vi "rsidr_core_global.vi"() -> ()   [LabVIEW 2020, in "Rohde&Schwarz RTx Oscilloscopes.lvlib"]
doc: "This Global variable contains driver's:\n- Attributes\n- Range Tables\n- Repeated Capabilities"
uses:
  Rohde&Schwarz RTx Oscilloscopes.lvlib
  type_Input_Format_Attribute.ctl
  type_Input_Format_RangeTable.ctl
  type_Input_Format_RepCap.ctl
  rsidr_core.lvlib
panel:
  in  "Repeated Capabilities":T1[](array[typedef])=[{"repCapName"="Channel", "indetifiers"=["CH0", "CH1", "CH2", "CH3", "CH4", "CHExt"], "cmdValues"=["", "1", "2", "3", "4", "5"]}, {"repCapName"="Measurement", "indetifiers"=["M1", "M2", "M3", "M4", "M5", "M6", "M7", "M8"], "cmdValues"=["1", "2", "3", "4", "5", "6", "7", "8"]}, {"repCapName"="Math", "indetifiers"=["MA1", "MA2", "MA3", "MA4", "MA5"], "cmdValues"=["1", "2", "3", "4", "5"]}, {"repCapName"="ReferenceWfm", "indetifiers"=["RW1", "RW2", "RW3", "RW4"], "cmdValues"=["1", "2", "3", "4"]}, {"repCapName"="SerialBus", "indetifiers"=["SB1", "SB2", "SB3", "SB4"], "cmdValues"=["1", "2", "3", "4"]}, {"repCapName"="Cursor", "indetifiers"=["Cur1", "Cur2", "Cur3"], "cmdValues"=["1", "2", "3"]}, {"repCapName"="ResultNumber", "indetifiers"=["Res1", "Res2", "Res3", "Res4", "Res5", "Res6", "Res7", "Res8", "Res9", "Res10", "Res11", "Res12", "Res13", "Res14", "Res15", "Res16", "Res17", "Res18", "Res19", "Res20", "Res21", "Res22", "Res23", "Res24", "Res25", "Res26", "Res27", "Res28", "Res29", "Res30", "Res31", "Res32", "Res33", "Res34", "Res35", "Res36", "Res37", "Res38", "Res39", "Res40"], "cmdValues"=["1", "2", "3", "4", "5", "6", "7", "8", "9", "10", "11", "12", "13", "14", "15", "16", "17", "18", "19", "20", "21", "22", "23", "24", "25", "26", "27", "28", "29", "30", "31", "32", "33", "34", "35", "36", "37", "38", "39", "40"]}, {"repCapName"="Gate", "indetifiers"=["Gate1", "Gate2", "Gate3"], "cmdValues"=["1", "2", "3"]}, {"repCapName"="OnOffResult", "indetifiers"=["OOR1", "OOR2", "OOR3"], "cmdValues"=["1", "2", "3"]}, {"repCapName"="SourceNumber", "indetifiers"=["S1", "S2", "S3", "S4"], "cmdValues"=["1", "2", "3", "4"]}, {"repCapName"="TDMChannel", "indetifiers"=["TDM0", "TDM1", "TDM2", "TDM3", "TDM4", "TDM5", "TDM6", "TDM7", "TDM8"], "cmdValues"=["", "1", "2", "3", "4", "5", "6", "7", "8"]}, {"repCapName"="Digital", "indetifiers"=["D0", "D1", "D2", "D3", "D4", "D5", "D6", "D7", "D8", "D9", "D10", "D11", "D12", "D13", "D14", "D15"], "cmdValues"=["0", "1", "2", "3", "4", "5", "6", "7", "8", "9", "10", "11", "12", "13", "14", "15"]}, {"repCapName"="DigitalVoltmeter", "indetifiers"=["DVM1", "DVM2", "DVM3", "DVM4"], "cmdValues"=["1", "2", "3", "4"]}, {"repCapName"="CursorLine", "indetifiers"=["CursorLine1", "CursorLine2"], "cmdValues"=["1", "2"]}, {"repCapName"="Logic", "indetifiers"=["Logic1", "Logic2"], "cmdValues"=["1", "2"]}, {"repCapName"="OutputPin", "indetifiers"=["P0", "P1", "P2", "P3"], "cmdValues"=["0", "1", "2", "3"]}, {"repCapName"="ProfilePoint", "indetifiers"=["Point1", "Point2", "Point3", "Point4", "Point5", "Point6", "Point7", "Point8", "Point9", "Point10", "Point11", "Point12", "Point13", "Point14", "Point15", "Point16"], "cmdValues"=["1", "2", "3", "4", "5", "6", "7", "8", "9", "10", "11", "12", "13", "14", "15", "16"]}, {"repCapName"="BodeMarker", "indetifiers"=["BodeMark1", "BodeMark2"], "cmdValues"=["1", "2"]}, {"repCapName"="ParallelLine", "indetifiers"=["Bit0", "Bit1", "Bit2", "Bit3", "Bit4", "Bit5", "Bit6", "Bit7", "Bit8", "Bit9", "Bit10", "Bit11", "Bit12", "Bit13", "Bit14", "Bit15"], "cmdValues"=["0", "1", "2", "3", "4", "5", "6", "7", "8", "9", "10", "11", "12", "13", "14", "15"]}]
  in  "Range Tables":T2[](array[typedef])=[{"Type"=0, "Name"="rsrtx_rngHorzScale", "Entries"=[{"Name"="", "Value 1"=1e-09, "Value 2"=50.0, "Command"=""}]}, {"Type"=0, "Name"="rsrtx_rngHorzAcquisitionTime", "Entries"=[{"Name"="", "Value 1"=2.5e-10, "Value 2"=500.0, "Command"=""}]}, {"Type"=0, "Name"="rsrtx_rngAcquisitionStartTime", "Entries"=[{"Name"="", "Value 1"=-500.0, "Value 2"=500.0, "Command"=""}]}, {"Type"=0, "Name"="rsrtx_rngHorzReference", "Entries"=[{"Name"="", "Value 1"=8.33, "Value 2"=91.67, "Command"=""}]}, {"Type"=2, "Name"="rsrtx_rngSampleMode", "Entries"=[{"Name"="Real Time", "Value 1"=0.0, "Value 2"=0.0, "Command"="RTIM"}, {"Name"="Equivalent Time", "Value 1"=1.0, "Value 2"=0.0, "Command"="ETIM"}]}, {"Type"=2, "Name"="rsrtx_rngWaveformArithmetics", "Entries"=[{"Name"="Off", "Value 1"=0.0, "Value 2"=0.0, "Command"="OFF"}, {"Name"="Envelope", "Value 1"=1.0, "Value 2"=0.0, "Command"="ENV"}, {"Name"="Average", "Value 1"=2.0, "Value 2"=0.0, "Command"="AVER"}, {"Name"="Smooth", "Value 1"=3.0, "Value 2"=0.0, "Command"="SMO"}, {"Name"="Filter", "Value 1"=4.0, "Value 2"=0.0, "Command"="FILT"}]}, {"Type"=2, "Name"="rsrtx_rngVerticalCoupling", "Entries"=[{"Name"="AC", "Value 1"=0.0, "Value 2"=0.0, "Command"="AC"}, {"Name"="DC 50 Ohm", "Value 1"=1.0, "Value 2"=0.0, "Command"="DC"}, {"Name"="DC 1 MOhm", "Value 1"=2.0, "Value 2"=0.0, "Command"="DCL"}, {"Name"="AC 1 MOhm", "Value 1"=3.0, "Value 2"=0.0, "Command"="ACL"}, {"Name"="Ground", "Value 1"=4.0, "Value 2"=0.0, "Command"="GND"}]}, {"Type"=2, "Name"="rsrtx_rngChannelBWLimit", "Entries"=[{"Name"="Full", "Value 1"=0.0, "Value 2"=0.0, "Command"="FULL"}, {"Name"="400 MHz", "Value 1"=1.0, "Value 2"=0.0, "Command"="B400"}, {"Name"="200 MHz", "Value 1"=2.0, "Value 2"=0.0, "Command"="B200"}, {"Name"="20 MHz", "Value 1"=3.0, "Value 2"=0.0, "Command"="B20"}]}, {"Type"=2, "Name"="rsrtx_rngTriggerSource", "Entries"=[{"Name"="Channel 1", "Value 1"=1.0, "Value 2"=0.0, "Command"="CH1"}, {"Name"="Channel 2", "Value 1"=2.0, "Value 2"=0.0, "Command"="CH2"}, {"Name"="Channel 3", "Value 1"=3.0, "Value 2"=0.0, "Command"="CH3"}, {"Name"="Channel 4", "Value 1"=4.0, "Value 2"=0.0, "Command"="CH4"}, {"Name"="External Trigger Input", "Value 1"=5.0, "Value 2"=0.0, "Command"="EXT"}, {"Name"="AC Line", "Value 1"=6.0, "Value 2"=0.0, "Command"="LINE"}, {"Name"="Serial Bus 1", "Value 1"=7.0, "Value 2"=0.0, "Command"="SBUS1"}, {"Name"="Serial Bus 2", "Value 1"=8.0, "Value 2"=0.0, "Command"="SBUS2"}, {"Name"="Serial Bus 3", "Value 1"=9.0, "Value 2"=0.0, "Command"="SBUS3"}, {"Name"="Serial Bus 4", "Value 1"=10.0, "Value 2"=0.0, "Command"="SBUS4"}, {"Name"="Digital 0", "Value 1"=11.0, "Value 2"=0.0, "Command"="D0"}, {"Name"="Digital 1", "Value 1"=12.0, "Value 2"=0.0, "Command"="D1"}, {"Name"="Digital 2", "Value 1"=13.0, "Value 2"=0.0, "Command"="D2"}, {"Name"="Digital 3", "Value 1"=14.0, "Value 2"=0.0, "Command"="D3"}, {"Name"="Digital 4", "Value 1"=15.0, "Value 2"=0.0, "Command"="D4"}, {"Name"="Digital 5", "Value 1"=16.0, "Value 2"=0.0, "Command"="D5"}, {"Name"="Digital 6", "Value 1"=17.0, "Value 2"=0.0, "Command"="D6"}, {"Name"="Digital 7", "Value 1"=18.0, "Value 2"=0.0, "Command"="D7"}, {"Name"="Digital 8", "Value 1"=19.0, "Value 2"=0.0, "Command"="D8"}, {"Name"="Digital 9", "Value 1"=20.0, "Value 2"=0.0, "Command"="D9"}, {"Name"="Digital 10", "Value 1"=21.0, "Value 2"=0.0, "Command"="D10"}, {"Name"="Digital 11", "Value 1"=22.0, "Value 2"=0.0, "Command"="D11"}, {"Name"="Digital 12", "Value 1"=23.0, "Value 2"=0.0, "Command"="D12"}, {"Name"="Digital 13", "Value 1"=24.0, "Value 2"=0.0, "Command"="D13"}, {"Name"="Digital 14", "Value 1"=25.0, "Value 2"=0.0, "Command"="D14"}, {"Name"="Digital 15", "Value 1"=26.0, "Value 2"=0.0, "Command"="D15"}]}, {"Type"=0, "Name"="rsrtx_rngTriggerLevel", "Entries"=[{"Name"="", "Value 1"=-10.0, "Value 2"=10.0, "Command"=""}]}, {"Type"=2, "Name"="rsrtx_rngTriggerSlope", "Entries"=[{"Name"="Rising Edge", "Value 1"=0.0, "Value 2"=0.0, "Command"="POS"}, {"Name"="Falling Edge", "Value 1"=1.0, "Value 2"=0.0, "Command"="NEG"}, {"Name"="Either", "Value 1"=2.0, "Value 2"=0.0, "Command"="EITH"}]}, {"Type"=2, "Name"="rsrtx_rngPolarity", "Entries"=[{"Name"="Negative", "Value 1"=0.0, "Value 2"=0.0, "Command"="NEG"}, {"Name"="Positive", "Value 1"=1.0, "Value 2"=0.0, "Command"="POS"}]}, {"Type"=2, "Name"="rsrtx_rngWidthCondition", "Entries"=[{"Name"="Shorter", "Value 1"=0.0, "Value 2"=0.0, "Command"="SHOR"}, {"Name"="Longer", "Value 1"=1.0, "Value 2"=0.0, "Command"="LONG"}, {"Name"="Within", "Value 1"=2.0, "Value 2"=0.0, "Command"="WITH"}, {"Name"="Outside", "Value 1"=3.0, "Value 2"=0.0, "Command"="OUTS"}]}, {"Type"=0, "Name"="rsrtx_rngLineNumber", "Entries"=[{"Name"="", "Value 1"=1.0, "Value 2"=1125.0, "Command"=""}]}, {"Type"=2, "Name"="rsrtx_rngTVTriggerEvent", "Entries"=[{"Name"="Even", "Value 1"=0.0, "Value 2"=0.0, "Command"="EVEN"}, {"Name"="Odd", "Value 1"=1.0, "Value 2"=0.0, "Command"="ODD"}, {"Name"="All", "Value 1"=2.0, "Value 2"=0.0, "Command"="ALL"}, {"Name"="Line", "Value 1"=3.0, "Value 2"=0.0, "Command"="LINE"}, {"Name"="All Line", "Value 1"=4.0, "Value 2"=0.0, "Command"="ALIN"}]}, {"Type"=2, "Name"="rsrtx_rngCursorFunction", "Entries"=[{"Name"="Horizontal", "Value 1"=0.0, "Value 2"=0.0, "Command"="HOR"}, {"Name"="Vertical", "Value 1"=1.0, "Value 2"=0.0, "Command"="VERT"}, {"Name"="Paired", "Value 1"=2.0, "Value 2"=0.0, "Command"="PAIR"}, {"Name"="H Ratio", "Value 1"=3.0, "Value 2"=0.0, "Command"="HRAT"}, {"Name"="V Ratio", "Value 1"=4.0, "Value 2"=0.0, "Command"="VRAT"}, {"Name"="Count Positive", "Value 1"=5.0, "Value 2"=0.0, "Command"="PPC"}, {"Name"="Count Negative", "Value 1"=6.0, "Value 2"=0.0, "Command"="NPC"}, {"Name"="Count Rising", "Value 1"=7.0, "Value 2"=0.0, "Command"="REC"}, {"Name"="Count Falling", "Value 1"=8.0, "Value 2"=0.0, "Command"="FEC"}, {"Name"="Mean", "Value 1"=9.0, "Value 2"=0.0, "Command"="MEAN"}, {"Name"="Root Mean", "Value 1"=10.0, "Value 2"=0.0, "Command"="RMS"}, {"Name"="Rise", "Value 1"=11.0, "Value 2"=0.0, "Command"="RTIM"}, {"Name"="Fall", "Value 1"=12.0, "Value 2"=0.0, "Command"="FTIM"}, {"Name"="Peak", "Value 1"=13.0, "Value 2"=0.0, "Command"="PEAK"}, {"Name"="Upper Peak", "Value 1"=14.0, "Value 2"=0.0, "Command"="UPE"}, {"Name"="Lower Peak", "Value 1"=15.0, "Value 2"=0.0, "Command"="LPE"}, {"Name"="Burst", "Value 1"=16.0, "Value 2"=0.0, "Command"="BWID"}, {"Name"="Horizontal Vertical", "Value 1"=17.0, "Value 2"=0.0, "Command"="HVER"}]}, {"Type"=0, "Name"="rsrtx_rngCursorXPosition", "Entries"=[{"Name"="", "Value 1"=0.0, "Value 2"=500.0, "Command"=""}]}, {"Type"=0, "Name"="rsrtx_rngCursorYPosition", "Entries"=[{"Name"="", "Value 1"=-50.0, "Value 2"=50.0, "Command"=""}]}, {"Type"=0, "Name"="rsrtx_rngPct", "Entries"=[{"Name"="", "Value 1"=0.0, "Value 2"=100.0, "Command"=""}]}, {"Type"=2, "Name"="rsrtx_rngXRatioMeasurementUnit", "Entries"=[{"Name"="Floating", "Value 1"=0.0, "Value 2"=0.0, "Command"="RAT"}, {"Name"="Percent", "Value 1"=1.0, "Value 2"=0.0, "Command"="PCT"}, {"Name"="Degree", "Value 1"=2.0, "Value 2"=0.0, "Command"="GRD"}, {"Name"="Radian", "Value 1"=3.0, "Value 2"=0.0, "Command"="PI"}]}, {"Type"=2, "Name"="rsrtx_rngYRatioMeasurementUnit", "Entries"=[{"Name"="Floating", "Value 1"=0.0, "Value 2"=0.0, "Command"="RAT"}, {"Name"="Percent", "Value 1"=1.0, "Value 2"=0.0, "Command"="PCT"}]}, {"Type"=2, "Name"="rsrtx_rngInterpolation", "Entries"=[{"Name"="sin(x)/x", "Value 1"=0.0, "Value 2"=0.0, "Command"="SINX"}, {"Name"="Linear", "Value 1"=1.0, "Value 2"=0.0, "Command"="LIN"}, {"Name"="Sample/Hold", "Value 1"=2.0, "Value 2"=0.0, "Command"="SMHD"}]}, {"Type"=2, "Name"="rsrtx_rngMeasurementCategory", "Entries"=[{"Name"="Amplitude And Time", "Value 1"=0.0, "Value 2"=0.0, "Command"="AMPT"}]}, {"Type"=2, "Name"="rsrtx_rngFFTWindowType", "Entries"=[{"Name"="Rectangular", "Value 1"=0.0, "Value 2"=0.0, "Command"="RECT"}, {"Name"="Hamming", "Value 1"=1.0, "Value 2"=0.0, "Command"="HAMM"}, {"Name"="Hann", "Value 1"=2.0, "Value 2"=0.0, "Command"="HANN"}, {"Name"="Blackman", "Value 1"=3.0, "Value 2"=0.0, "Command"="BLAC"}, {"Name"="Flat Top", "Value 1"=4.0, "Value 2"=0.0, "Command"="FLAT"}]}, {"Type"=0, "Name"="rsrtx_rngRBW", "Entries"=[{"Name"="", "Value 1"=100.0, "Value 2"=2000000.0, "Command"=""}]}, {"Type"=0, "Name"="rsrtx_rngRBWRatio", "Entries"=[{"Name"="", "Value 1"=1024.0, "Value 2"=32768.0, "Command"=""}]}, {"Type"=2, "Name"="rsrtx_rngProtocolI2CFrameState", "Entries"=[{"Name"="Ok", "Value 1"=0.0, "Value 2"=0.0, "Command"="OK"}, {"Name"="Incomplete", "Value 1"=1.0, "Value 2"=0.0, "Command"="INC"}, {"Name"="Unexpected Stop", "Value 1"=2.0, "Value 2"=0.0, "Command"="UNEX"}, {"Name"="Insufficient", "Value 1"=3.0, "Value 2"=0.0, "Command"="INS"}, {"Name"="Add", "Value 1"=4.0, "Value 2"=0.0, "Command"="ADD"}]}, {"Type"=2, "Name"="rsrtx_rngProtocolAckBit", "Entries"=[{"Name"="Either", "Value 1"=0.0, "Value 2"=0.0, "Command"="EITH"}, {"Name"="Ack", "Value 1"=1.0, "Value 2"=0.0, "Command"="ACK"}, {"Name"="NAck", "Value 1"=2.0, "Value 2"=0.0, "Command"="NACK"}, {"Name"="Missing", "Value 1"=3.0, "Value 2"=0.0, "Command"="INC"}]}, {"Type"=2, "Name"="rsrtx_rngProtocolSPIBitOrder", "Entries"=[{"Name"="Most significant bit", "Value 1"=0.0, "Value 2"=0.0, "Command"="MSBF"}, {"Name"="Least significant bit", "Value 1"=1.0, "Value 2"=0.0, "Command"="LSBF"}]}, {"Type"=0, "Name"="rsrtx_rngProtocolSPIWordLength", "Entries"=[{"Name"="", "Value 1"=4.0, "Value 2"=32.0, "Command"=""}]}, {"Type"=2, "Name"="rsrtx_rngAudioSource", "Entries"=[{"Name"="Channel 1", "Value 1"=1.0, "Value 2"=0.0, "Command"="CH1"}, {"Name"="Channel 2", "Value 1"=2.0, "Value 2"=0.0, "Command"="CH2"}, {"Name"="Channel 3", "Value 1"=3.0, "Value 2"=0.0, "Command"="CH3"}, {"Name"="Channel 4", "Value 1"=4.0, "Value 2"=0.0, "Command"="CH4"}, {"Name"="Digital Channel 0", "Value 1"=5.0, "Value 2"=0.0, "Command"="D0"}, {"Name"="Digital Channel 1", "Value 1"=6.0, "Value 2"=0.0, "Command"="D1"}, {"Name"="Digital Channel 2", "Value 1"=7.0, "Value 2"=0.0, "Command"="D2"}, {"Name"="Digital Channel 3", "Value 1"=8.0, "Value 2"=0.0, "Command"="D3"}, {"Name"="Digital Channel 4", "Value 1"=9.0, "Value 2"=0.0, "Command"="D4"}, {"Name"="Digital Channel 5", "Value 1"=10.0, "Value 2"=0.0, "Command"="D5"}, {"Name"="Digital Channel 6", "Value 1"=11.0, "Value 2"=0.0, "Command"="D6"}, {"Name"="Digital Channel 7", "Value 1"=12.0, "Value 2"=0.0, "Command"="D7"}, {"Name"="Digital Channel 8", "Value 1"=13.0, "Value 2"=0.0, "Command"="D8"}, {"Name"="Digital Channel 9", "Value 1"=14.0, "Value 2"=0.0, "Command"="D9"}, {"Name"="Digital Channel 10", "Value 1"=15.0, "Value 2"=0.0, "Command"="D10"}, {"Name"="Digital Channel 11", "Value 1"=16.0, "Value 2"=0.0, "Command"="D11"}, {"Name"="Digital Channel 12", "Value 1"=17.0, "Value 2"=0.0, "Command"="D12"}, {"Name"="Digital Channel 13", "Value 1"=18.0, "Value 2"=0.0, "Command"="D13"}, {"Name"="Digital Channel 14", "Value 1"=19.0, "Value 2"=0.0, "Command"="D14"}, {"Name"="Digital Channel 15", "Value 1"=20.0, "Value 2"=0.0, "Command"="D15"}]}, {"Type"=2, "Name"="rsrtx_rngSPIChipSelectSource", "Entries"=[{"Name"="Channel 1", "Value 1"=1.0, "Value 2"=0.0, "Command"="CH1"}, {"Name"="Channel 2", "Value 1"=2.0, "Value 2"=0.0, "Command"="CH2"}, {"Name"="Channel 3", "Value 1"=3.0, "Value 2"=0.0, "Command"="CH3"}, {"Name"="Channel 4", "Value 1"=4.0, "Value 2"=0.0, "Command"="CH4"}, {"Name"="Digital Channel 0", "Value 1"=5.0, "Value 2"=0.0, "Command"="D0"}, {"Name"="Digital Channel 1", "Value 1"=6.0, "Value 2"=0.0, "Command"="D1"}, {"Name"="Digital Channel 2", "Value 1"=7.0, "Value 2"=0.0, "Command"="D2"}, {"Name"="Digital Channel 3", "Value 1"=8.0, "Value 2"=0.0, "Command"="D3"}, {"Name"="Digital Channel 4", "Value 1"=9.0, "Value 2"=0.0, "Command"="D4"}, {"Name"="Digital Channel 5", "Value 1"=10.0, "Value 2"=0.0, "Command"="D5"}, {"Name"="Digital Channel 6", "Value 1"=11.0, "Value 2"=0.0, "Command"="D6"}, {"Name"="Digital Channel 7", "Value 1"=12.0, "Value 2"=0.0, "Command"="D7"}, {"Name"="Digital Channel 8", "Value 1"=13.0, "Value 2"=0.0, "Command"="D8"}, {"Name"="Digital Channel 9", "Value 1"=14.0, "Value 2"=0.0, "Command"="D9"}, {"Name"="Digital Channel 10", "Value 1"=15.0, "Value 2"=0.0, "Command"="D10"}, {"Name"="Digital Channel 11", "Value 1"=16.0, "Value 2"=0.0, "Command"="D11"}, {"Name"="Digital Channel 12", "Value 1"=17.0, "Value 2"=0.0, "Command"="D12"}, {"Name"="Digital Channel 13", "Value 1"=18.0, "Value 2"=0.0, "Command"="D13"}, {"Name"="Digital Channel 14", "Value 1"=19.0, "Value 2"=0.0, "Command"="D14"}, {"Name"="Digital Channel 15", "Value 1"=20.0, "Value 2"=0.0, "Command"="D15"}]}, {"Type"=2, "Name"="rsrtx_rngMOSISource", "Entries"=[{"Name"="Channel 1", "Value 1"=1.0, "Value 2"=0.0, "Command"="CH1"}, {"Name"="Channel 2", "Value 1"=2.0, "Value 2"=0.0, "Command"="CH2"}, {"Name"="Channel 3", "Value 1"=3.0, "Value 2"=0.0, "Command"="CH3"}, {"Name"="Channel 4", "Value 1"=4.0, "Value 2"=0.0, "Command"="CH4"}, {"Name"="Digital Channel 0", "Value 1"=5.0, "Value 2"=0.0, "Command"="D0"}, {"Name"="Digital Channel 1", "Value 1"=6.0, "Value 2"=0.0, "Command"="D1"}, {"Name"="Digital Channel 2", "Value 1"=7.0, "Value 2"=0.0, "Command"="D2"}, {"Name"="Digital Channel 3", "Value 1"=8.0, "Value 2"=0.0, "Command"="D3"}, {"Name"="Digital Channel 4", "Value 1"=9.0, "Value 2"=0.0, "Command"="D4"}, {"Name"="Digital Channel 5", "Value 1"=10.0, "Value 2"=0.0, "Command"="D5"}, {"Name"="Digital Channel 6", "Value 1"=11.0, "Value 2"=0.0, "Command"="D6"}, {"Name"="Digital Channel 7", "Value 1"=12.0, "Value 2"=0.0, "Command"="D7"}, {"Name"="Digital Channel 8", "Value 1"=13.0, "Value 2"=0.0, "Command"="D8"}, {"Name"="Digital Channel 9", "Value 1"=14.0, "Value 2"=0.0, "Command"="D9"}, {"Name"="Digital Channel 10", "Value 1"=15.0, "Value 2"=0.0, "Command"="D10"}, {"Name"="Digital Channel 11", "Value 1"=16.0, "Value 2"=0.0, "Command"="D11"}, {"Name"="Digital Channel 12", "Value 1"=17.0, "Value 2"=0.0, "Command"="D12"}, {"Name"="Digital Channel 13", "Value 1"=18.0, "Value 2"=0.0, "Command"="D13"}, {"Name"="Digital Channel 14", "Value 1"=19.0, "Value 2"=0.0, "Command"="D14"}, {"Name"="Digital Channel 15", "Value 1"=20.0, "Value 2"=0.0, "Command"="D15"}]}, {"Type"=2, "Name"="rsrtx_rngMISOSource", "Entries"=[{"Name"="None", "Value 1"=0.0, "Value 2"=0.0, "Command"="NONE"}, {"Name"="Channel 1", "Value 1"=1.0, "Value 2"=0.0, "Command"="CH1"}, {"Name"="Channel 2", "Value 1"=2.0, "Value 2"=0.0, "Command"="CH2"}, {"Name"="Channel 3", "Value 1"=3.0, "Value 2"=0.0, "Command"="CH3"}, {"Name"="Channel 4", "Value 1"=4.0, "Value 2"=0.0, "Command"="CH4"}, {"Name"="Digital Channel 0", "Value 1"=5.0, "Value 2"=0.0, "Command"="D0"}, {"Name"="Digital Channel 1", "Value 1"=6.0, "Value 2"=0.0, "Command"="D1"}, {"Name"="Digital Channel 2", "Value 1"=7.0, "Value 2"=0.0, "Command"="D2"}, {"Name"="Digital Channel 3", "Value 1"=8.0, "Value 2"=0.0, "Command"="D3"}, {"Name"="Digital Channel 4", "Value 1"=9.0, "Value 2"=0.0, "Command"="D4"}, {"Name"="Digital Channel 5", "Value 1"=10.0, "Value 2"=0.0, "Command"="D5"}, {"Name"="Digital Channel 6", "Value 1"=11.0, "Value 2"=0.0, "Command"="D6"}, {"Name"="Digital Channel 7", "Value 1"=12.0, "Value 2"=0.0, "Command"="D7"}, {"Name"="Digital Channel 8", "Value 1"=13.0, "Value 2"=0.0, "Command"="D8"}, {"Name"="Digital Channel 9", "Value 1"=14.0, "Value 2"=0.0, "Command"="D9"}, {"Name"="Digital Channel 10", "Value 1"=15.0, "Value 2"=0.0, "Command"="D10"}, {"Name"="Digital Channel 11", "Value 1"=16.0, "Value 2"=0.0, "Command"="D11"}, {"Name"="Digital Channel 12", "Value 1"=17.0, "Value 2"=0.0, "Command"="D12"}, {"Name"="Digital Channel 13", "Value 1"=18.0, "Value 2"=0.0, "Command"="D13"}, {"Name"="Digital Channel 14", "Value 1"=19.0, "Value 2"=0.0, "Command"="D14"}, {"Name"="Digital Channel 15", "Value 1"=20.0, "Value 2"=0.0, "Command"="D15"}]}, {"Type"=2, "Name"="rsrtx_rngProtocolSPIPolarity", "Entries"=[{"Name"="Low active (low = 1)", "Value 1"=0.0, "Value 2"=0.0, "Command"="NEG"}, {"Name"="High active (high = 1)", "Value 1"=1.0, "Value 2"=0.0, "Command"="POS"}]}, {"Type"=2, "Name"="rsrtx_rngProtocolSPIFrameState", "Entries"=[{"Name"="OK", "Value 1"=0.0, "Value 2"=0.0, "Command"="OK"}, {"Name"="Incomplete first", "Value 1"=1.0, "Value 2"=0.0, "Command"="INCF"}, {"Name"="Incomplete last", "Value 1"=2.0, "Value 2"=0.0, "Command"="INCL"}, {"Name"="Insufficient", "Value 1"=3.0, "Value 2"=0.0, "Command"="INS"}, {"Name"="Void", "Value 1"=4.0, "Value 2"=0.0, "Command"="VOID"}]}, {"Type"=2, "Name"="rsrtx_rngUARTSource", "Entries"=[{"Name"="Channel 1", "Value 1"=1.0, "Value 2"=0.0, "Command"="CH1"}, {"Name"="Channel 2", "Value 1"=2.0, "Value 2"=0.0, "Command"="CH2"}, {"Name"="Channel 3", "Value 1"=3.0, "Value 2"=0.0, "Command"="CH3"}, {"Name"="Channel 4", "Value 1"=4.0, "Value 2"=0.0, "Command"="CH4"}, {"Name"="Digital Channel 0", "Value 1"=5.0, "Value 2"=0.0, "Command"="D0"}, {"Name"="Digital Channel 1", "Value 1"=6.0, "Value 2"=0.0, "Command"="D1"}, {"Name"="Digital Channel 2", "Value 1"=7.0, "Value 2"=0.0, "Command"="D2"}, {"Name"="Digital Channel 3", "Value 1"=8.0, "Value 2"=0.0, "Command"="D3"}, {"Name"="Digital Channel 4", "Value 1"=9.0, "Value 2"=0.0, "Command"="D4"}, {"Name"="Digital Channel 5", "Value 1"=10.0, "Value 2"=0.0, "Command"="D5"}, {"Name"="Digital Channel 6", "Value 1"=11.0, "Value 2"=0.0, "Command"="D6"}, {"Name"="Digital Channel 7", "Value 1"=12.0, "Value 2"=0.0, "Command"="D7"}, {"Name"="Digital Channel 8", "Value 1"=13.0, "Value 2"=0.0, "Command"="D8"}, {"Name"="Digital Channel 9", "Value 1"=14.0, "Value 2"=0.0, "Command"="D9"}, {"Name"="Digital Channel 10", "Value 1"=15.0, "Value 2"=0.0, "Command"="D10"}, {"Name"="Digital Channel 11", "Value 1"=16.0, "Value 2"=0.0, "Command"="D11"}, {"Name"="Digital Channel 12", "Value 1"=17.0, "Value 2"=0.0, "Command"="D12"}, {"Name"="Digital Channel 13", "Value 1"=18.0, "Value 2"=0.0, "Command"="D13"}, {"Name"="Digital Channel 14", "Value 1"=19.0, "Value 2"=0.0, "Command"="D14"}, {"Name"="Digital Channel 15", "Value 1"=20.0, "Value 2"=0.0, "Command"="D15"}]}, {"Type"=2, "Name"="rsrtx_rngUARTTxSource", "Entries"=[{"Name"="None", "Value 1"=0.0, "Value 2"=0.0, "Command"="NONE"}, {"Name"="Channel 1", "Value 1"=1.0, "Value 2"=0.0, "Command"="CH1"}, {"Name"="Channel 2", "Value 1"=2.0, "Value 2"=0.0, "Command"="CH2"}, {"Name"="Channel 3", "Value 1"=3.0, "Value 2"=0.0, "Command"="CH3"}, {"Name"="Channel 4", "Value 1"=4.0, "Value 2"=0.0, "Command"="CH4"}, {"Name"="Digital Channel 0", "Value 1"=5.0, "Value 2"=0.0, "Command"="D0"}, {"Name"="Digital Channel 1", "Value 1"=6.0, "Value 2"=0.0, "Command"="D1"}, {"Name"="Digital Channel 2", "Value 1"=7.0, "Value 2"=0.0, "Command"="D2"}, {"Name"="Digital Channel 3", "Value 1"=8.0, "Value 2"=0.0, "Command"="D3"}, {"Name"="Digital Channel 4", "Value 1"=9.0, "Value 2"=0.0, "Command"="D4"}, {"Name"="Digital Channel 5", "Value 1"=10.0, "Value 2"=0.0, "Command"="D5"}, {"Name"="Digital Channel 6", "Value 1"=11.0, "Value 2"=0.0, "Command"="D6"}, {"Name"="Digital Channel 7", "Value 1"=12.0, "Value 2"=0.0, "Command"="D7"}, {"Name"="Digital Channel 8", "Value 1"=13.0, "Value 2"=0.0, "Command"="D8"}, {"Name"="Digital Channel 9", "Value 1"=14.0, "Value 2"=0.0, "Command"="D9"}, {"Name"="Digital Channel 10", "Value 1"=15.0, "Value 2"=0.0, "Command"="D10"}, {"Name"="Digital Channel 11", "Value 1"=16.0, "Value 2"=0.0, "Command"="D11"}, {"Name"="Digital Channel 12", "Value 1"=17.0, "Value 2"=0.0, "Command"="D12"}, {"Name"="Digital Channel 13", "Value 1"=18.0, "Value 2"=0.0, "Command"="D13"}, {"Name"="Digital Channel 14", "Value 1"=19.0, "Value 2"=0.0, "Command"="D14"}, {"Name"="Digital Channel 15", "Value 1"=20.0, "Value 2"=0.0, "Command"="D15"}]}, {"Type"=2, "Name"="rsrtx_rngProtocolUARTParity", "Entries"=[{"Name"="None", "Value 1"=0.0, "Value 2"=0.0, "Command"="NONE"}, {"Name"="Odd", "Value 1"=1.0, "Value 2"=0.0, "Command"="ODD"}, {"Name"="Even", "Value 1"=2.0, "Value 2"=0.0, "Command"="EVEN"}]}, {"Type"=2, "Name"="rsrtx_rngProtocolUARTStopBits", "Entries"=[{"Name"="B1", "Value 1"=0.0, "Value 2"=0.0, "Command"="B1"}, {"Name"="B15", "Value 1"=1.0, "Value 2"=0.0, "Command"="B1_5"}, {"Name"="B2", "Value 1"=2.0, "Value 2"=0.0, "Command"="B2"}]}, {"Type"=2, "Name"="rsrtx_rngProtocolUARTTriggerType", "Entries"=[{"Name"="Burst start", "Value 1"=0.0, "Value 2"=0.0, "Command"="BST"}, {"Name"="Start bit", "Value 1"=1.0, "Value 2"=0.0, "Command"="SBIT"}, {"Name"="N-th symbol", "Value 1"=2.0, "Value 2"=0.0, "Command"="NTHS"}, {"Name"="Symbol", "Value 1"=3.0, "Value 2"=0.0, "Command"="SYMB"}, {"Name"="Pattern", "Value 1"=4.0, "Value 2"=0.0, "Command"="PATT"}, {"Name"="Parity error", "Value 1"=5.0, "Value 2"=0.0, "Command"="PRER"}, {"Name"="Stop bit error", "Value 1"=6.0, "Value 2"=0.0, "Command"="SPER"}, {"Name"="Break", "Value 1"=7.0, "Value 2"=0.0, "Command"="BRE"}, {"Name"="Frame Error", "Value 1"=8.0, "Value 2"=0.0, "Command"="FERR"}]}, {"Type"=2, "Name"="rsrtx_rngSignalStyle", "Entries"=[{"Name"="Vectors", "Value 1"=0.0, "Value 2"=0.0, "Command"="VECT"}, {"Name"="Dots", "Value 1"=1.0, "Value 2"=0.0, "Command"="DOTS"}]}, {"Type"=2, "Name"="rsrtx_rngHardcopyDeviceOrientation", "Entries"=[{"Name"="Portrait", "Value 1"=0.0, "Value 2"=0.0, "Command"="PORT"}, {"Name"="Landscape", "Value 1"=1.0, "Value 2"=0.0, "Command"="LAND"}]}, {"Type"=2, "Name"="rsrtx_rngWaveformParameter", "Entries"=[{"Name"="Channel 1", "Value 1"=1.0, "Value 2"=0.0, "Command"="CH1"}, {"Name"="Channel 2", "Value 1"=2.0, "Value 2"=0.0, "Command"="CH2"}, {"Name"="Channel 3", "Value 1"=3.0, "Value 2"=0.0, "Command"="CH3"}, {"Name"="Channel 4", "Value 1"=4.0, "Value 2"=0.0, "Command"="CH4"}, {"Name"="Math Waveform 1", "Value 1"=5.0, "Value 2"=0.0, "Command"="MA1"}, {"Name"="Math Waveform 2", "Value 1"=6.0, "Value 2"=0.0, "Command"="MA2"}, {"Name"="Math Waveform 3", "Value 1"=7.0, "Value 2"=0.0, "Command"="MA3"}, {"Name"="Math Waveform 4", "Value 1"=8.0, "Value 2"=0.0, "Command"="MA4"}, {"Name"="Math Waveform 5", "Value 1"=9.0, "Value 2"=0.0, "Command"="MA5"}, {"Name"="Reference Waveform 1", "Value 1"=10.0, "Value 2"=0.0, "Command"="RE1"}, {"Name"="Reference Waveform 2", "Value 1"=11.0, "Value 2"=0.0, "Command"="RE2"}, {"Name"="Reference Waveform 3", "Value 1"=12.0, "Value 2"=0.0, "Command"="RE3"}, {"Name"="Reference Waveform 4", "Value 1"=13.0, "Value 2"=0.0, "Command"="RE4"}, {"Name"="Digital 0", "Value 1"=14.0, "Value 2"=0.0, "Command"="D0"}, {"Name"="Digital 1", "Value 1"=15.0, "Value 2"=0.0, "Command"="D1"}, {"Name"="Digital 2", "Value 1"=16.0, "Value 2"=0.0, "Command"="D2"}, {"Name"="Digital 3", "Value 1"=17.0, "Value 2"=0.0, "Command"="D3"}, {"Name"="Digital 4", "Value 1"=18.0, "Value 2"=0.0, "Command"="D4"}, {"Name"="Digital 5", "Value 1"=19.0, "Value 2"=0.0, "Command"="D5"}, {"Name"="Digital 6", "Value 1"=20.0, "Value 2"=0.0, "Command"="D6"}, {"Name"="Digital 7", "Value 1"=21.0, "Value 2"=0.0, "Command"="D7"}, {"Name"="Digital 8", "Value 1"=22.0, "Value 2"=0.0, "Command"="D8"}, {"Name"="Digital 9", "Value 1"=23.0, "Value 2"=0.0, "Command"="D9"}, {"Name"="Digital 10", "Value 1"=24.0, "Value 2"=0.0, "Command"="D10"}, {"Name"="Digital11", "Value 1"=25.0, "Value 2"=0.0, "Command"="D11"}, {"Name"="Digital 12", "Value 1"=26.0, "Value 2"=0.0, "Command"="D12"}, {"Name"="Digital 13", "Value 1"=27.0, "Value 2"=0.0, "Command"="D13"}, {"Name"="Digital 14", "Value 1"=28.0, "Value 2"=0.0, "Command"="D14"}, {"Name"="Digital 15", "Value 1"=29.0, "Value 2"=0.0, "Command"="D15"}, {"Name"="Digital 70", "Value 1"=30.0, "Value 2"=0.0, "Command"="D70"}, {"Name"="Digital 158", "Value 1"=31.0, "Value 2"=0.0, "Command"="D158"}, {"Name"="Spectrum", "Value 1"=32.0, "Value 2"=0.0, "Command"="SPEC"}, {"Name"="XY2", "Value 1"=33.0, "Value 2"=0.0, "Command"="XY2"}, {"Name"="Minimum Hold", "Value 1"=34.0, "Value 2"=0.0, "Command"="MINH"}, {"Name"="Maximum Hold", "Value 1"=35.0, "Value 2"=0.0, "Command"="MAXH"}, {"Name"="Average", "Value 1"=36.0, "Value 2"=0.0, "Command"="AVER"}, {"Name"="QMA", "Value 1"=37.0, "Value 2"=0.0, "Command"="QMA"}, {"Name"="XY1", "Value 1"=38.0, "Value 2"=0.0, "Command"="XY1"}]}, {"Type"=0, "Name"="rsrtx_rngAveragingSpectrums", "Entries"=[{"Name"="", "Value 1"=2.0, "Value 2"=512.0, "Command"=""}]}, {"Type"=2, "Name"="rsrtx_rngColorBrightness", "Entries"=[{"Name"="Normal", "Value 1"=0.0, "Value 2"=0.0, "Command"="NORM"}, {"Name"="Inverse", "Value 1"=1.0, "Value 2"=0.0, "Command"="INV"}, {"Name"="Frequenct Color", "Value 1"=2.0, "Value 2"=0.0, "Command"="FCOL"}, {"Name"="Inverse Color", "Value 1"=3.0, "Value 2"=0.0, "Command"="IFC"}]}, {"Type"=2, "Name"="rsrtx_rngDiagramMode", "Entries"=[{"Name"="YT", "Value 1"=0.0, "Value 2"=0.0, "Command"="YT"}, {"Name"="XY", "Value 1"=1.0, "Value 2"=0.0, "Command"="XY"}]}, {"Type"=2, "Name"="rsrtx_rngLanguage", "Entries"=[{"Name"="English", "Value 1"=0.0, "Value 2"=0.0, "Command"="ENGL"}, {"Name"="German", "Value 1"=1.0, "Value 2"=0.0, "Command"="GERM"}, {"Name"="French", "Value 1"=2.0, "Value 2"=0.0, "Command"="FREN"}, {"Name"="Spanish", "Value 1"=3.0, "Value 2"=0.0, "Command"="SPAN"}, {"Name"="Russian", "Value 1"=4.0, "Value 2"=0.0, "Command"="RUSS"}, {"Name"="Simplified Chinese", "Value 1"=5.0, "Value 2"=0.0, "Command"="SCH"}, {"Name"="Traditional Chinese", "Value 1"=6.0, "Value 2"=0.0, "Command"="TCH"}, {"Name"="Japanese", "Value 1"=7.0, "Value 2"=0.0, "Command"="JAP"}, {"Name"="Korean", "Value 1"=8.0, "Value 2"=0.0, "Command"="KOR"}, {"Name"="Italian", "Value 1"=9.0, "Value 2"=0.0, "Command"="ITAL"}, {"Name"="Portuguese", "Value 1"=10.0, "Value 2"=0.0, "Command"="PORT"}, {"Name"="Czech", "Value 1"=11.0, "Value 2"=0.0, "Command"="CZEC"}, {"Name"="Polish", "Value 1"=12.0, "Value 2"=0.0, "Command"="POL"}]}, {"Type"=2, "Name"="rsrtx_rngGridStyle", "Entries"=[{"Name"="Lines", "Value 1"=0.0, "Value 2"=0.0, "Command"="LIN"}, {"Name"="Cross", "Value 1"=1.0, "Value 2"=0.0, "Command"="RET"}, {"Name"="None", "Value 1"=2.0, "Value 2"=0.0, "Command"="NONE"}]}, {"Type"=2, "Name"="rsrtx_rngSource", "Entries"=[{"Name"="Channel 1", "Value 1"=1.0, "Value 2"=0.0, "Command"="CH1"}, {"Name"="Channel 2", "Value 1"=2.0, "Value 2"=0.0, "Command"="CH2"}, {"Name"="Channel 3", "Value 1"=3.0, "Value 2"=0.0, "Command"="CH3"}, {"Name"="Channel 4", "Value 1"=4.0, "Value 2"=0.0, "Command"="CH4"}]}, {"Type"=2, "Name"="rsrtx_rngXY2Source", "Entries"=[{"Name"="None", "Value 1"=0.0, "Value 2"=0.0, "Command"="NONE"}, {"Name"="Channel 1", "Value 1"=1.0, "Value 2"=0.0, "Command"="CH1"}, {"Name"="Channel 2", "Value 1"=2.0, "Value 2"=0.0, "Command"="CH2"}, {"Name"="Channel 3", "Value 1"=3.0, "Value 2"=0.0, "Command"="CH3"}, {"Name"="Channel 4", "Value 1"=4.0, "Value 2"=0.0, "Command"="CH4"}]}, {"Type"=2, "Name"="rsrtx_rngIntensityMode", "Entries"=[{"Name"="Analog", "Value 1"=0.0, "Value 2"=0.0, "Command"="ANAL"}, {"Name"="Digital", "Value 1"=1.0, "Value 2"=0.0, "Command"="DIG"}, {"Name"="Off", "Value 1"=2.0, "Value 2"=0.0, "Command"="OFF"}]}, {"Type"=0, "Name"="rsrtx_rngIntensityTreshold", "Entries"=[{"Name"="", "Value 1"=-10.0, "Value 2"=0.0, "Command"=""}]}, {"Type"=2, "Name"="rsrtx_rngHardcopyDevice", "Entries"=[{"Name"="Mem", "Value 1"=0.0, "Value 2"=0.0, "Command"="MMEM"}, {"Name"="Print", "Value 1"=1.0, "Value 2"=0.0, "Command"="SYST:COMM:PRIN"}]}, {"Type"=2, "Name"="rsrtx_rngHardcopyDeviceLang", "Entries"=[{"Name"="BMP", "Value 1"=1.0, "Value 2"=0.0, "Command"="BMP"}, {"Name"="PNG", "Value 1"=0.0, "Value 2"=0.0, "Command"="PNG"}, {"Name"="GDI", "Value 1"=2.0, "Value 2"=0.0, "Command"="GDI"}, {"Name"="GIF", "Value 1"=3.0, "Value 2"=0.0, "Command"="GIF"}]}, {"Type"=2, "Name"="rsrtx_rngMaskCondition", "Entries"=[{"Name"="Run", "Value 1"=0.0, "Value 2"=0.0, "Command"="RUN"}, {"Name"="Stop", "Value 1"=1.0, "Value 2"=0.0, "Command"="STOP"}, {"Name"="Pause", "Value 1"=2.0, "Value 2"=0.0, "Command"="PAUS"}]}, {"Type"=2, "Name"="rsrtx_rngProbeButtonAction", "Entries"=[{"Name"="No Action", "Value 1"=0.0, "Value 2"=0.0, "Command"="NOAC"}, {"Name"="Continuous", "Value 1"=1.0, "Value 2"=0.0, "Command"="RCON"}, {"Name"="Run single", "Value 1"=2.0, "Value 2"=0.0, "Command"="RSIN"}, {"Name"="Autoset", "Value 1"=3.0, "Value 2"=0.0, "Command"="AUT"}]}, {"Type"=2, "Name"="rsrtx_rngTriggerCoupling", "Entries"=[{"Name"="Direct Current", "Value 1"=0.0, "Value 2"=0.0, "Command"="DC"}, {"Name"="Alternating Current", "Value 1"=1.0, "Value 2"=0.0, "Command"="AC"}, {"Name"="High frequency", "Value 1"=2.0, "Value 2"=0.0, "Command"="LFR"}]}, {"Type"=2, "Name"="rsrtx_rngProtocolI2CAccessBit", "Entries"=[{"Name"="Read", "Value 1"=1.0, "Value 2"=0.0, "Command"="READ"}, {"Name"="Write", "Value 1"=2.0, "Value 2"=0.0, "Command"="WRIT"}]}, {"Type"=2, "Name"="rsrtx_rngAddressLength", "Entries"=[{"Name"="Normal", "Value 1"=0.0, "Value 2"=0.0, "Command"="NORM"}, {"Name"="Extended", "Value 1"=1.0, "Value 2"=0.0, "Command"="EXT"}]}, {"Type"=2, "Name"="rsrtx_rngProtocolI2CTriggerType", "Entries"=[{"Name"="Start", "Value 1"=0.0, "Value 2"=0.0, "Command"="STAR"}, {"Name"="Restart", "Value 1"=1.0, "Value 2"=0.0, "Command"="REST"}, {"Name"="Stop", "Value 1"=2.0, "Value 2"=0.0, "Command"="STOP"}, {"Name"="Mode Missing", "Value 1"=3.0, "Value 2"=0.0, "Command"="MACK"}, {"Name"="Pattern", "Value 1"=4.0, "Value 2"=0.0, "Command"="PATT"}]}, {"Type"=2, "Name"="rsrtx_rngHysteresisMode", "Entries"=[{"Name"="Auto", "Value 1"=0.0, "Value 2"=0.0, "Command"="AUTO"}, {"Name"="Small", "Value 1"=1.0, "Value 2"=0.0, "Command"="SMAL"}, {"Name"="Medium", "Value 1"=2.0, "Value 2"=0.0, "Command"="MED"}, {"Name"="Large", "Value 1"=3.0, "Value 2"=0.0, "Command"="LARG"}, {"Name"="Manual", "Value 1"=4.0, "Value 2"=0.0, "Command"="MAN"}]}, {"Type"=2, "Name"="rsrtx_rngTriggerMode", "Entries"=[{"Name"="Auto", "Value 1"=0.0, "Value 2"=0.0, "Command"="AUTO"}, {"Name"="Normal", "Value 1"=1.0, "Value 2"=0.0, "Command"="NORM"}, {"Name"="Delay", "Value 1"=2.0, "Value 2"=0.0, "Command"="DEL"}, {"Name"="Events", "Value 1"=3.0, "Value 2"=0.0, "Command"="EVEN"}]}, {"Type"=2, "Name"="rsrtx_rngTriggerPatternFunction", "Entries"=[{"Name"="And", "Value 1"=0.0, "Value 2"=0.0, "Command"="AND"}, {"Name"="Or", "Value 1"=1.0, "Value 2"=0.0, "Command"="OR"}]}, {"Type"=2, "Name"="rsrtx_rngProtocolSPITriggerType", "Entries"=[{"Name"="Start", "Value 1"=0.0, "Value 2"=0.0, "Command"="BST"}, {"Name"="End", "Value 1"=1.0, "Value 2"=0.0, "Command"="BEND"}, {"Name"="nth", "Value 1"=2.0, "Value 2"=0.0, "Command"="NTHB"}, {"Name"="Pattern", "Value 1"=3.0, "Value 2"=0.0, "Command"="PATT"}]}, {"Type"=0, "Name"="rsrtx_rngFirstBitOffset", "Entries"=[{"Name"="", "Value 1"=0.0, "Value 2"=4095.0, "Command"=""}]}, {"Type"=0, "Name"="rsrtx_rngSPIWordLength", "Entries"=[{"Name"="", "Value 1"=1.0, "Value 2"=32.0, "Command"=""}]}, {"Type"=2, "Name"="rsrtx_rngTriggerType", "Entries"=[{"Name"="Edge", "Value 1"=0.0, "Value 2"=0.0, "Command"="EDGE"}, {"Name"="Width", "Value 1"=1.0, "Value 2"=0.0, "Command"="WIDT"}, {"Name"="Video", "Value 1"=2.0, "Value 2"=0.0, "Command"="TV"}, {"Name"="Pattern", "Value 1"=3.0, "Value 2"=0.0, "Command"="LOG"}, {"Name"="Bus", "Value 1"=4.0, "Value 2"=0.0, "Command"="BUS"}, {"Name"="Rise Time", "Value 1"=5.0, "Value 2"=0.0, "Command"="RIS"}, {"Name"="Runt", "Value 1"=6.0, "Value 2"=0.0, "Command"="RUNT"}, {"Name"="Line", "Value 1"=7.0, "Value 2"=0.0, "Command"="LINE"}]}, {"Type"=2, "Name"="rsrtx_rngTVStandard", "Entries"=[{"Name"="PAL", "Value 1"=0.0, "Value 2"=0.0, "Command"="PAL"}, {"Name"="NTSC", "Value 1"=1.0, "Value 2"=0.0, "Command"="NTSC"}, {"Name"="Secam", "Value 1"=2.0, "Value 2"=0.0, "Command"="SEC"}, {"Name"="PALM", "Value 1"=3.0, "Value 2"=0.0, "Command"="PALM"}, {"Name"="I576", "Value 1"=4.0, "Value 2"=0.0, "Command"="I576"}, {"Name"="P720", "Value 1"=5.0, "Value 2"=0.0, "Command"="P720"}, {"Name"="P1080", "Value 1"=6.0, "Value 2"=0.0, "Command"="P1080"}, {"Name"="I1080", "Value 1"=7.0, "Value 2"=0.0, "Command"="I1080"}]}, {"Type"=0, "Name"="rsrtx_rngUartLength", "Entries"=[{"Name"="", "Value 1"=1.0, "Value 2"=4.0, "Command"=""}]}, {"Type"=0, "Name"="rsrtx_rngTrgDelay", "Entries"=[{"Name"="", "Value 1"=2e-08, "Value 2"=6.87, "Command"=""}]}, {"Type"=2, "Name"="rsrtx_rngColorScheme", "Entries"=[{"Name"="Color", "Value 1"=0.0, "Value 2"=0.0, "Command"="COL"}, {"Name"="Grayscale", "Value 1"=1.0, "Value 2"=0.0, "Command"="GRAY"}, {"Name"="Inverted", "Value 1"=2.0, "Value 2"=0.0, "Command"="INV"}]}, {"Type"=2, "Name"="rsrtx_rngAcquisitionType", "Entries"=[{"Name"="Sample", "Value 1"=0.0, "Value 2"=0.0, "Command"="SAMP"}, {"Name"="Peak Detect", "Value 1"=1.0, "Value 2"=0.0, "Command"="PDET"}, {"Name"="High Resolution", "Value 1"=2.0, "Value 2"=0.0, "Command"="HRES"}]}, {"Type"=2, "Name"="rsrtx_rngAmplitudeTimeMeasurementType", "Entries"=[{"Name"="Frequency", "Value 1"=1.0, "Value 2"=0.0, "Command"="FREQ"}, {"Name"="Period", "Value 1"=2.0, "Value 2"=0.0, "Command"="PER"}, {"Name"="Peak Peak", "Value 1"=3.0, "Value 2"=0.0, "Command"="PEAK"}, {"Name"="Peak Upper", "Value 1"=4.0, "Value 2"=0.0, "Command"="UPE"}, {"Name"="Peak Lower", "Value 1"=5.0, "Value 2"=0.0, "Command"="LPE"}, {"Name"="Positive Pulses Count", "Value 1"=6.0, "Value 2"=0.0, "Command"="PPC"}, {"Name"="Negative Pulses Count", "Value 1"=7.0, "Value 2"=0.0, "Command"="NPC"}, {"Name"="Rising Edges Count", "Value 1"=8.0, "Value 2"=0.0, "Command"="REC"}, {"Name"="Falling Edges Count", "Value 1"=9.0, "Value 2"=0.0, "Command"="FEC"}, {"Name"="High", "Value 1"=10.0, "Value 2"=0.0, "Command"="HIGH"}, {"Name"="Low", "Value 1"=11.0, "Value 2"=0.0, "Command"="LOW"}, {"Name"="Amplitude", "Value 1"=12.0, "Value 2"=0.0, "Command"="AMPL"}, {"Name"="Mean Value", "Value 1"=13.0, "Value 2"=0.0, "Command"="MEAN"}, {"Name"="RMS Value", "Value 1"=14.0, "Value 2"=0.0, "Command"="RMS"}, {"Name"="Rise Time", "Value 1"=15.0, "Value 2"=0.0, "Command"="RTIM"}, {"Name"="Falling Time", "Value 1"=16.0, "Value 2"=0.0, "Command"="FTIM"}, {"Name"="Duty Cycle Positive", "Value 1"=17.0, "Value 2"=0.0, "Command"="PDCY"}, {"Name"="Duty Cycle Negative", "Value 1"=18.0, "Value 2"=0.0, "Command"="NDCY"}, {"Name"="Pulse Width Positive", "Value 1"=19.0, "Value 2"=0.0, "Command"="PPW"}, {"Name"="Pulse Width Negative", "Value 1"=20.0, "Value 2"=0.0, "Command"="NPW"}, {"Name"="Cycle Mean", "Value 1"=21.0, "Value 2"=0.0, "Command"="CYCM"}, {"Name"="Cycle RMS", "Value 1"=22.0, "Value 2"=0.0, "Command"="CYCR"}, {"Name"="Standard Deviation", "Value 1"=23.0, "Value 2"=0.0, "Command"="STDD"}, {"Name"="Trigger Frequency", "Value 1"=24.0, "Value 2"=0.0, "Command"="TFR"}, {"Name"="Trigger Period", "Value 1"=25.0, "Value 2"=0.0, "Command"="TPER"}, {"Name"="Delay", "Value 1"=26.0, "Value 2"=0.0, "Command"="DEL"}, {"Name"="Phase", "Value 1"=27.0, "Value 2"=0.0, "Command"="PHAS"}, {"Name"="Burst Width", "Value 1"=28.0, "Value 2"=0.0, "Command"="BWID"}, {"Name"="Cycle Standard Deviation", "Value 1"=29.0, "Value 2"=0.0, "Command"="CYCS"}, {"Name"="Positive Overshoot", "Value 1"=30.0, "Value 2"=0.0, "Command"="POV"}, {"Name"="Negative Overshoot", "Value 1"=31.0, "Value 2"=0.0, "Command"="NOV"}, {"Name"="Trigger B Frequency", "Value 1"=32.0, "Value 2"=0.0, "Command"="TBFR"}, {"Name"="Trigger B Period", "Value 1"=33.0, "Value 2"=0.0, "Command"="TBP"}, {"Name"="Slew Rate Rise", "Value 1"=34.0, "Value 2"=0.0, "Command"="SRR"}, {"Name"="Slew Rate Fall", "Value 1"=35.0, "Value 2"=0.0, "Command"="SRF"}, {"Name"="DTO Trigger", "Value 1"=36.0, "Value 2"=0.0, "Command"="DTOT"}]}, {"Type"=2, "Name"="rsrtx_rngProtocolType", "Entries"=[{"Name"="Parallel", "Value 1"=0.0, "Value 2"=0.0, "Command"="PAR"}, {"Name"="CParallel", "Value 1"=1.0, "Value 2"=0.0, "Command"="CPAR"}, {"Name"="I2C", "Value 1"=2.0, "Value 2"=0.0, "Command"="I2C"}, {"Name"="SPI", "Value 1"=3.0, "Value 2"=0.0, "Command"="SPI"}, {"Name"="SSPI", "Value 1"=4.0, "Value 2"=0.0, "Command"="SSPI"}, {"Name"="UART", "Value 1"=5.0, "Value 2"=0.0, "Command"="UART"}, {"Name"="CAN", "Value 1"=6.0, "Value 2"=0.0, "Command"="CAN"}, {"Name"="LIN", "Value 1"=7.0, "Value 2"=0.0, "Command"="LIN"}, {"Name"="Audio", "Value 1"=8.0, "Value 2"=0.0, "Command"="I2S"}, {"Name"="MILSTD", "Value 1"=9.0, "Value 2"=0.0, "Command"="MILS"}, {"Name"="ARINC429", "Value 1"=10.0, "Value 2"=0.0, "Command"="ARIN"}]}, {"Type"=2, "Name"="rsrtx_rngProtocolFormat", "Entries"=[{"Name"="Ascii", "Value 1"=0.0, "Value 2"=0.0, "Command"="ASC"}, {"Name"="Hexadecimal", "Value 1"=1.0, "Value 2"=0.0, "Command"="HEX"}, {"Name"="Binary", "Value 1"=2.0, "Value 2"=0.0, "Command"="BIN"}, {"Name"="Decimal", "Value 1"=3.0, "Value 2"=0.0, "Command"="DEC"}, {"Name"="Octal", "Value 1"=4.0, "Value 2"=0.0, "Command"="OCT"}]}, {"Type"=2, "Name"="rsrtx_rngProtocolHeight", "Entries"=[{"Name"="Small", "Value 1"=0.0, "Value 2"=0.0, "Command"="SMAL"}, {"Name"="Medium", "Value 1"=1.0, "Value 2"=0.0, "Command"="MED"}, {"Name"="Large", "Value 1"=2.0, "Value 2"=0.0, "Command"="LARG"}, {"Name"="DIV1", "Value 1"=3.0, "Value 2"=0.0, "Command"="DIV1"}, {"Name"="DIV2", "Value 1"=4.0, "Value 2"=0.0, "Command"="DIV2"}, {"Name"="DIV4", "Value 1"=5.0, "Value 2"=0.0, "Command"="DIV4"}, {"Name"="DIV8", "Value 1"=6.0, "Value 2"=0.0, "Command"="DIV8"}]}, {"Type"=0, "Name"="rsrtx_rngProtocolVertical", "Entries"=[{"Name"="", "Value 1"=-5.0, "Value 2"=5.0, "Command"=""}]}, {"Type"=0, "Name"="rsrtx_rngParallelBusAnalyzedLines", "Entries"=[{"Name"="", "Value 1"=1.0, "Value 2"=4.0, "Command"=""}]}, {"Type"=0, "Name"="rsrtx_rngProtocolBurstIdleTime", "Entries"=[{"Name"="", "Value 1"=1.6e-08, "Value 2"=0.000838832, "Command"=""}]}, {"Type"=0, "Name"="rsrtx_rngProtocolUARTWordLength", "Entries"=[{"Name"="", "Value 1"=5.0, "Value 2"=9.0, "Command"=""}]}, {"Type"=0, "Name"="rsrtx_rngProtocolUARTBitRate", "Entries"=[{"Name"="", "Value 1"=100.0, "Value 2"=78100000.0, "Command"=""}]}, {"Type"=0, "Name"="rsrtx_rngProtocolI2CPatternLength", "Entries"=[{"Name"="", "Value 1"=1.0, "Value 2"=3.0, "Command"=""}]}, {"Type"=0, "Name"="rsrtx_rngBckLight", "Entries"=[{"Name"="", "Value 1"=10.0, "Value 2"=100.0, "Command"=""}]}, {"Type"=2, "Name"="rsrtx_rngRelativeMode", "Entries"=[{"Name"="Ten", "Value 1"=0.0, "Value 2"=0.0, "Command"="TEN"}, {"Name"="Twenty", "Value 1"=1.0, "Value 2"=0.0, "Command"="TWEN"}, {"Name"="Five", "Value 1"=2.0, "Value 2"=0.0, "Command"="FIVE"}, {"Name"="User", "Value 1"=3.0, "Value 2"=0.0, "Command"="USER"}]}, {"Type"=2, "Name"="rsrtx_rngChannelPolarity", "Entries"=[{"Name"="Normal", "Value 1"=0.0, "Value 2"=0.0, "Command"="NORM"}, {"Name"="Inverted", "Value 1"=1.0, "Value 2"=0.0, "Command"="INV"}]}, {"Type"=2, "Name"="rsrtx_rngExternalTriggerCoupling", "Entries"=[{"Name"="AC", "Value 1"=0.0, "Value 2"=0.0, "Command"="AC"}, {"Name"="DC", "Value 1"=1.0, "Value 2"=0.0, "Command"="DC"}]}, {"Type"=0, "Name"="rsrtx_rngRelLevel", "Entries"=[{"Name"="", "Value 1"=0.0, "Value 2"=100.0, "Command"=""}]}, {"Type"=0, "Name"="rsrtx_rngMathVerticalScale", "Entries"=[{"Name"="", "Value 1"=-1e-24, "Value 2"=5e+25, "Command"=""}]}, {"Type"=2, "Name"="rsrtx_rngSearchCondition", "Entries"=[{"Name"="Edge", "Value 1"=0.0, "Value 2"=0.0, "Command"="EDGE"}, {"Name"="Width", "Value 1"=1.0, "Value 2"=0.0, "Command"="WIDT"}, {"Name"="Peak", "Value 1"=2.0, "Value 2"=0.0, "Command"="PEAK"}, {"Name"="Runt", "Value 1"=3.0, "Value 2"=0.0, "Command"="RUNT"}, {"Name"="Rise Time", "Value 1"=4.0, "Value 2"=0.0, "Command"="RTIM"}, {"Name"="Data2Clock", "Value 1"=5.0, "Value 2"=0.0, "Command"="DAT"}, {"Name"="Pattern", "Value 1"=6.0, "Value 2"=0.0, "Command"="PATT"}, {"Name"="Protocol", "Value 1"=7.0, "Value 2"=0.0, "Command"="PROT"}, {"Name"="Window", "Value 1"=8.0, "Value 2"=0.0, "Command"="WIND"}]}, {"Type"=2, "Name"="rsrtx_rngSearchSource", "Entries"=[{"Name"="Channel Waveform 1", "Value 1"=0.0, "Value 2"=0.0, "Command"="CH1"}, {"Name"="Channel Waveform 2", "Value 1"=1.0, "Value 2"=0.0, "Command"="CH2"}, {"Name"="Channel Waveform 3", "Value 1"=2.0, "Value 2"=0.0, "Command"="CH3"}, {"Name"="Channel Waveform 4", "Value 1"=3.0, "Value 2"=0.0, "Command"="CH4"}, {"Name"="Math Waveform 1", "Value 1"=4.0, "Value 2"=0.0, "Command"="MA1"}, {"Name"="Math Waveform 2", "Value 1"=5.0, "Value 2"=0.0, "Command"="MA2"}, {"Name"="Math Waveform 3", "Value 1"=6.0, "Value 2"=0.0, "Command"="MA3"}, {"Name"="Math Waveform 
